vi "告警接口-告警存储-交互.vi"(11 "map in":T1) -> (3 "data":T2)   [LabVIEW 2016, in "Alarm interface.lvlib"]
uses:
  Alarm interface.lvlib
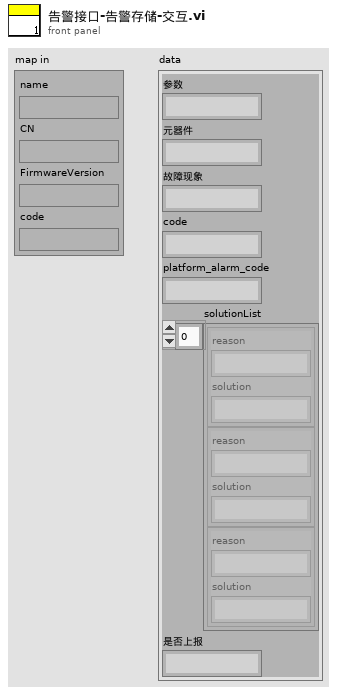
[diagram p1: front panel]
types:
  T1 = typedef "Alarm interface.lvlib/map in.ctl" = cluster{"name":string, "CN":string, "FirmwareVersion":string, "code":string}
  T2 = typedef "Alarm interface.lvlib/报警短信语音交互.ctl" = cluster{"参数":string, "元器件":string, "故障现象":string, "code":string, "platform_alarm_code":string, "solutionList":cluster{"reason":string, "solution":string}[], "是否上报":string}
  T3 = typedef "Alarm interface.lvlib/map out.ctl" = cluster{"componentParent":string, "componentName":string, "equipVersion":string, "ipcAlarmCode":string, "faultPhenomenon":string}
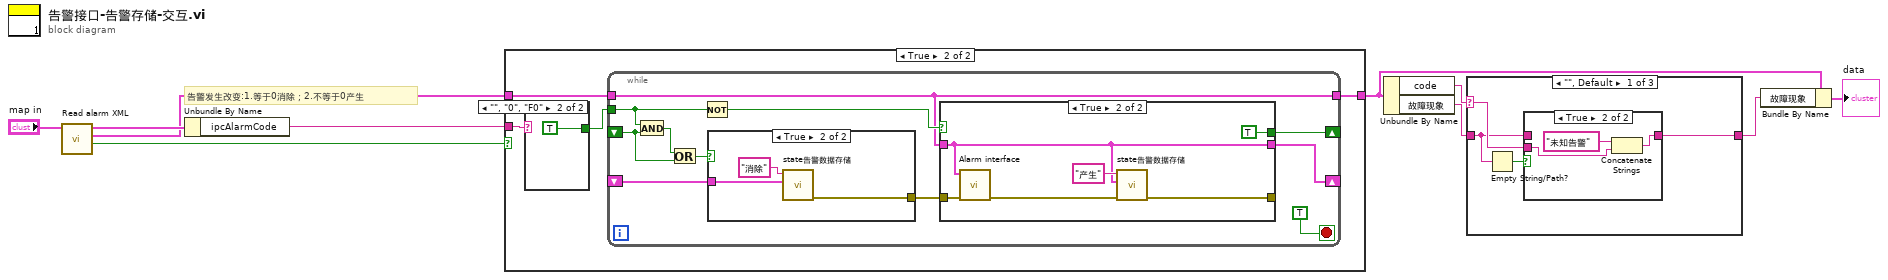
[diagram p0: block diagram]
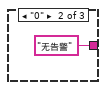
[diagram p7: hidden frame]
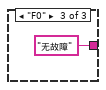
[diagram p8: hidden frame]
diagram:
  # "告警发生改变:1.等于0消除；2.不等于0产生"
  n1 = call "Read alarm XML.vi"("map in"="map in") -> ("map out"=w10:T3, "data"=w2:T2, "change?"=w4:bool)  [unwired: 7 in]
  n2 = Unbundle By Name(w10) -> ("ipcAlarmCode"=w3:string)
  n3 = case shown="True" w4 {
    tunnel: w3 -> [_ w15]
    tunnel: w2 -> [w11 w13]
    tunnel: [w11 w12] -> w1
    frame False {
    }
    frame True {
      n4 = case shown="\"\", \"0\", \"F0\"" w15 {
        tunnel: [_ TRUE] -> w14
        frame Default {
        }
        frame "", "0", "F0" {
        }
      }
      n5 = while {
        shift-right: [w24] -> _
        shift-left: _ -> [w18]
        tunnel: w14 -> [w20]
        tunnel: w13 -> [w21]
        shift-right: [w22] -> _
        shift-left: _ -> [w23]
        tunnel: [w21] -> w12
        stop <- TRUE stop-if-true
        n6 = And(x=w20, y=w18) -> (x .and. y?=w19:bool)
        n7 = Or(x=w19, y=w18) -> (x .or. y?=w17:bool)
        n8 = Not(x=w20) -> (.not. x?=w26:bool)
        n9 = case shown="True" w17 {
          tunnel: [_ w36] -> w25
          tunnel: w23 -> [_ w35]
          frame False {
          }
          frame True {
            n10 = call "state告警数据存储.vi"("data"=w35, "state"="消除") -> ("错误输出"=w36:errorcluster)  [unwired: 9 in]
          }
        }
        n11 = case shown="True" w26 {
          tunnel: w25 -> [_ w34]
          tunnel: w21 -> [w28 w29]
          tunnel: [_ w31] -> _
          tunnel: [_ TRUE] -> w24
          tunnel: [w28 w29] -> w22
          frame False {
          }
          frame True {
            n12 = call "Alarm interface.vi"("错误输入（无错误）"=w34, "簇"=w29) -> ("错误输出"=w32:errorcluster)  [unwired: 9 in]
            n13 = call "state告警数据存储.vi"("错误输入（无错误）"=w32, "data"=w29, "state"="产生") -> ("错误输出"=w31:errorcluster)  [unwired: 8 in]
          }
        }
      }
    }
  }
  n14 = Unbundle By Name(w1) -> ("code"=w9:string, "故障现象"=w8:string)
  n15 = case shown="\"\", Default" w9 {
    selector: w9 -> [w40 _ _]
    tunnel: w8 -> [w38 _ _]
    tunnel: [w39 "无告警" "无故障"] -> w7
    frame "", Default {
      n16 = Empty String/Path?(string/path=w38) -> (empty?=w41:bool)
      n17 = case shown="True" w41 {
        tunnel: w40 -> [_ w44]
        tunnel: [w42 w43] -> w39
        tunnel: w38 -> [w42 _]
        frame False {
        }
        frame True {
          n18 = Concatenate Strings("未知告警", w44) -> (w43:string)
        }
      }
    }
    frame "0" {
    }
    frame "F0" {
    }
  }
  n19 = Bundle By Name(cluster=w1, "故障现象"=w7) -> (→"data":T2)
